vi "Sim_Diff_Drive_Globals.vi"() -> ()   [LabVIEW 2019]
panel:
  in  "IMU angle(degrees)":dbl
  in  "Left_Wheel_Velocity":dbl
  in  "Right_Wheel_Velocity":dbl
  in  "Right_Wheel_Position":dbl
  in  "Left_Wheel_Position":dbl
  in  "Left_Wheel_Force_Input":dbl
  in  "Right_Wheel_Force_Input":dbl
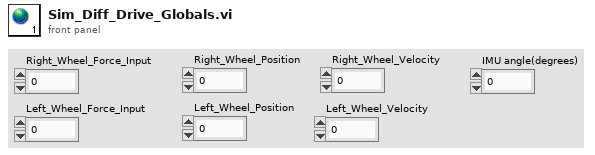
[diagram p1: front panel]
diagram:
